vi "Create New File.vi"(8 "error in (no error)":errorcluster) -> (0 "error out":errorcluster, 3 "Created File":refnum<file>)   [LabVIEW 2020]
uses:
  Type Definitions/Writeable Drives.ctl
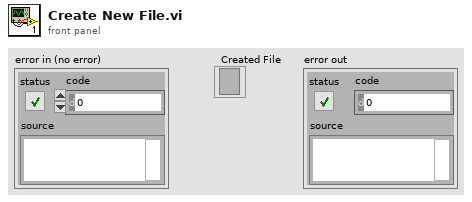
[diagram p1: front panel]
types:
  T1 = typedef "Writeable Drives.ctl" = cluster{"USB/SD Drives":path[], "Hard Drives":path[]}
  T2 = typedef "LVDateTimeRec.ctl" = cluster{"fractional second":dbl, "second":i32, "minute":i32, "hour":i32, "day of month":i32, "month":i32, "year":i32, "day of week":i32, "day of year":i32, "DST":i32}
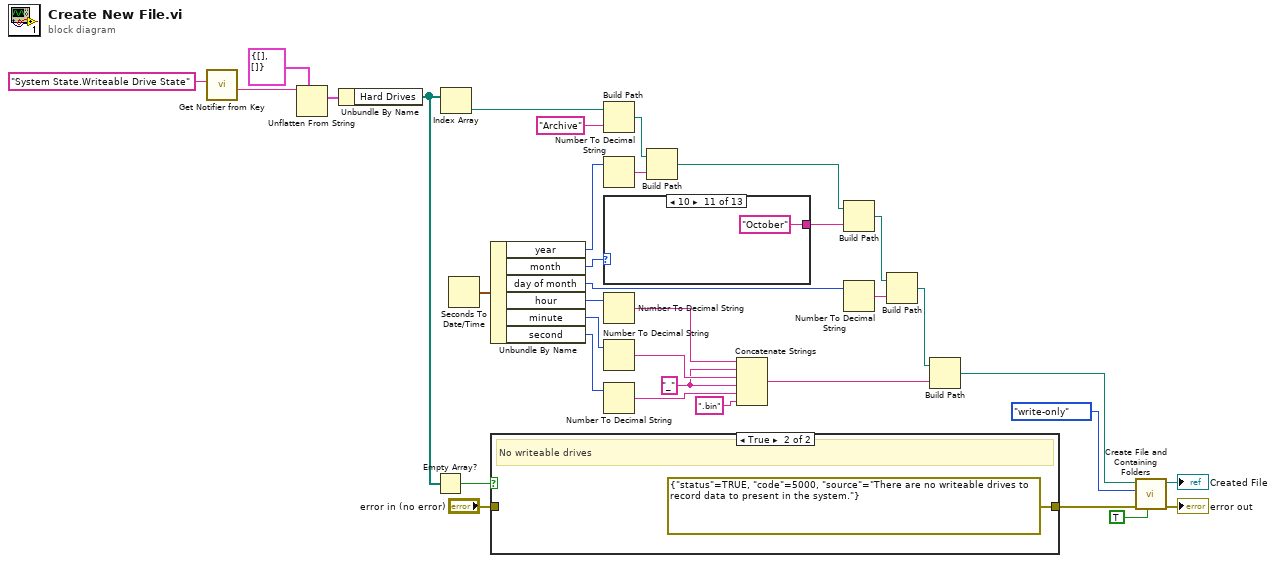
[diagram p0: block diagram]
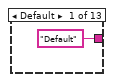
[diagram p3: hidden frame]
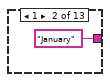
[diagram p4: hidden frame]
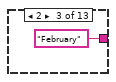
[diagram p5: hidden frame]
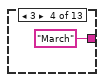
[diagram p6: hidden frame]
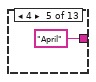
[diagram p7: hidden frame]
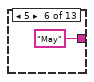
[diagram p8: hidden frame]
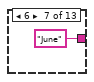
[diagram p9: hidden frame]
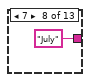
[diagram p10: hidden frame]
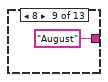
[diagram p11: hidden frame]
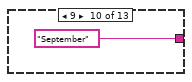
[diagram p12: hidden frame]
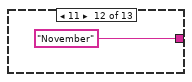
[diagram p13: hidden frame]
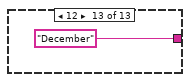
[diagram p14: hidden frame]
diagram:
  w8 = "_" ("string")
  n1 = call "Get Notifier from Key.vi"("Notifier Key"="System State.Writeable Drive State") -> ("Payload"=w27:string)  [unwired: 8 in, 2 out]
  n2 = Unflatten From String(type=T1 {"USB/SD Drives"=[], "Hard Drives"=[]} ("Writeable Drives"), binary string=w27) -> (value=w30:T1)  [unwired: 3 in, 2 out]
  n3 = Unbundle By Name(w30) -> ("Hard Drives"=w31:path[])
  n4 = Empty Array?(array=w31) -> (empty?=w1:bool)
  n5 = Index Array(array=w31) -> (element=w2:path)  [unwired: 1 in]
  n6 = Seconds To Date/Time() -> (date time rec=w3:T2)  [unwired: 2 in]
  n7 = Unbundle By Name(w3) -> ("year"=w16:i32, "month"=w17:i32, "day of month"=w15:i32, "hour"=w14:i32, "minute"=w13:i32, "second"=w12:i32)
  n8 = case shown="True" w1 {
    tunnel: [w36 errorcluster {"status"=TRUE, "code"=5000, "source"="There are no writeable drives to record data to present in the system."} ("error out")] -> w34
    tunnel: "error in (no error)" -> [w36 _]
    frame False {
      # "Writeable drives"
    }
    frame True {
      # "No writeable drives"
    }
  }
  n9 = Build Path(base path=w2, name or relative path="Archive") -> (appended path=w26:path)
  n10 = Number To Decimal String(number=w16) -> (decimal integer string=w25:string)  [unwired: 1 in]
  n11 = case shown="10" w17 {
    tunnel: ["Default" "January" "February" "March" "April" "May" "June" "July" "August" "September" "October" "November" "December"] -> w21
    frame Default {
    }
    frame 1 {
    }
    frame 2 {
    }
    frame 3 {
    }
    frame 4 {
    }
    frame 5 {
    }
    frame 6 {
    }
    frame 7 {
    }
    frame 8 {
    }
    frame 9 {
    }
    frame 10 {
    }
    frame 11 {
    }
    frame 12 {
    }
  }
  n12 = Number To Decimal String(number=w14) -> (decimal integer string=w10:string)  [unwired: 1 in]
  n13 = Number To Decimal String(number=w13) -> (decimal integer string=w9:string)  [unwired: 1 in]
  n14 = Number To Decimal String(number=w12) -> (decimal integer string=w7:string)  [unwired: 1 in]
  n15 = Build Path(base path=w26, name or relative path=w25) -> (appended path=w20:path)
  n16 = Concatenate Strings(w10, w8, w9, w8, w7, ".bin" ("string")) -> (w5:string)
  n17 = Build Path(base path=w20, name or relative path=w21) -> (appended path=w22:path)
  n18 = Number To Decimal String(number=w15) -> (decimal integer string=w23:string)  [unwired: 1 in]
  n19 = Build Path(base path=w22, name or relative path=w23) -> (appended path=w24:path)
  n20 = Build Path(base path=w24, name or relative path=w5) -> (appended path=w18:path)
  n21 = call <vilib>:"Create File and Containing Folders.vi"("disable buffering (F)"=TRUE, "error in (no error)"=w34, "access"=enum16{"read/write", "read-only", "write-only"}."write-only", "file path"=w18) -> ("error out"=→"error out":errorcluster, "refnum out"=→"Created File":refnum<file>)  [unwired: 6 in]
